vi "get_number_of_position_feedback_samples_for_delay_correction.vi"(8 "error in (no error)":errorcluster, 11 "TrajectoryDL091126GenericVoxel in":refnum<class "TrajectoryDL091126GenericVoxel.lvclass">) -> (0 "error out":errorcluster, 2 "number of pixels required":i32, 3 "TrajectoryDL091126GenericVoxel out":refnum<class "TrajectoryDL091126GenericVoxel.lvclass">)   [LabVIEW 2010, in "TrajectoryDL091126GenericVoxel.lvclass"]
uses:
  TrajectoryDL091126GenericVoxel.lvclass
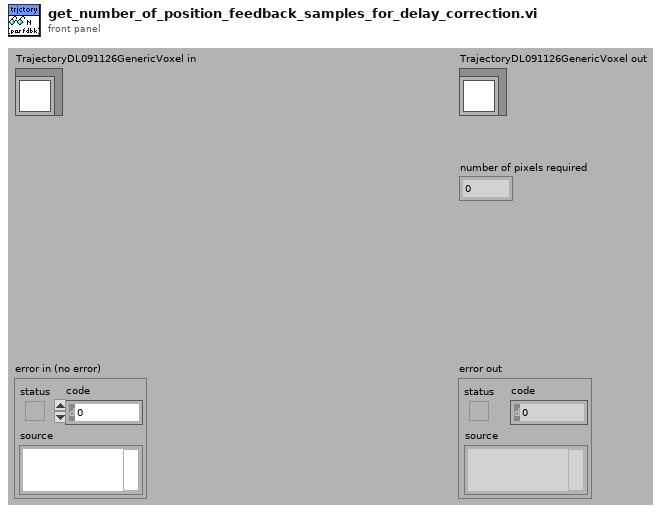
[diagram p1: front panel]
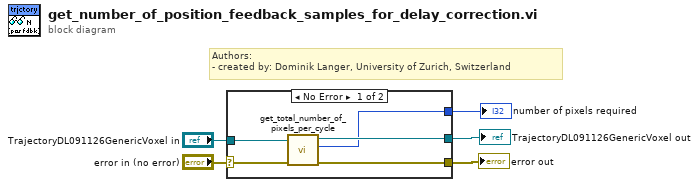
[diagram p0: block diagram]
diagram:
  # "Authors: \n- created by: Dominik Langer, University of Zurich, Switzerland"
  n1 = case shown="No Error" "error in (no error)" {
    selector: "error in (no error)" -> [w10 w12]
    tunnel: [w9 w12] -> w4
    tunnel: [w7 w11] -> w2
    tunnel: "TrajectoryDL091126GenericVoxel in" -> [w8 w11]
    tunnel: [w6 _] -> w1
    frame No Error {
      n2 = call-dynamic "get_total_number_of_pixels_per_cycle.vi"("error in (no error)"=w10, "GenericTrajectory in"=w8) -> ("error out"=w9:errorcluster, "total number of pixels per cycle"=w6:i32, "GenericTrajectory out"=w7:refnum<class "TrajectoryDL091126GenericVoxel.lvclass">)  [unwired: 7 in]
    }
    frame Error {
    }
  }
  "error out" <- w4
  "TrajectoryDL091126GenericVoxel out" <- w2
  "number of pixels required" <- w1
